vi "Send_Basic_Trajectory.vi"(8 "error in (no error)":errorcluster, 10 "TrajectoryPoint":T1) -> (0 "error out":errorcluster)   [LabVIEW 2019]
uses:
  <vilib>/Utility/error.llb/Error Cluster From Error Code.vi
  <vilib>/ErrorRing/Error Ring.xnode
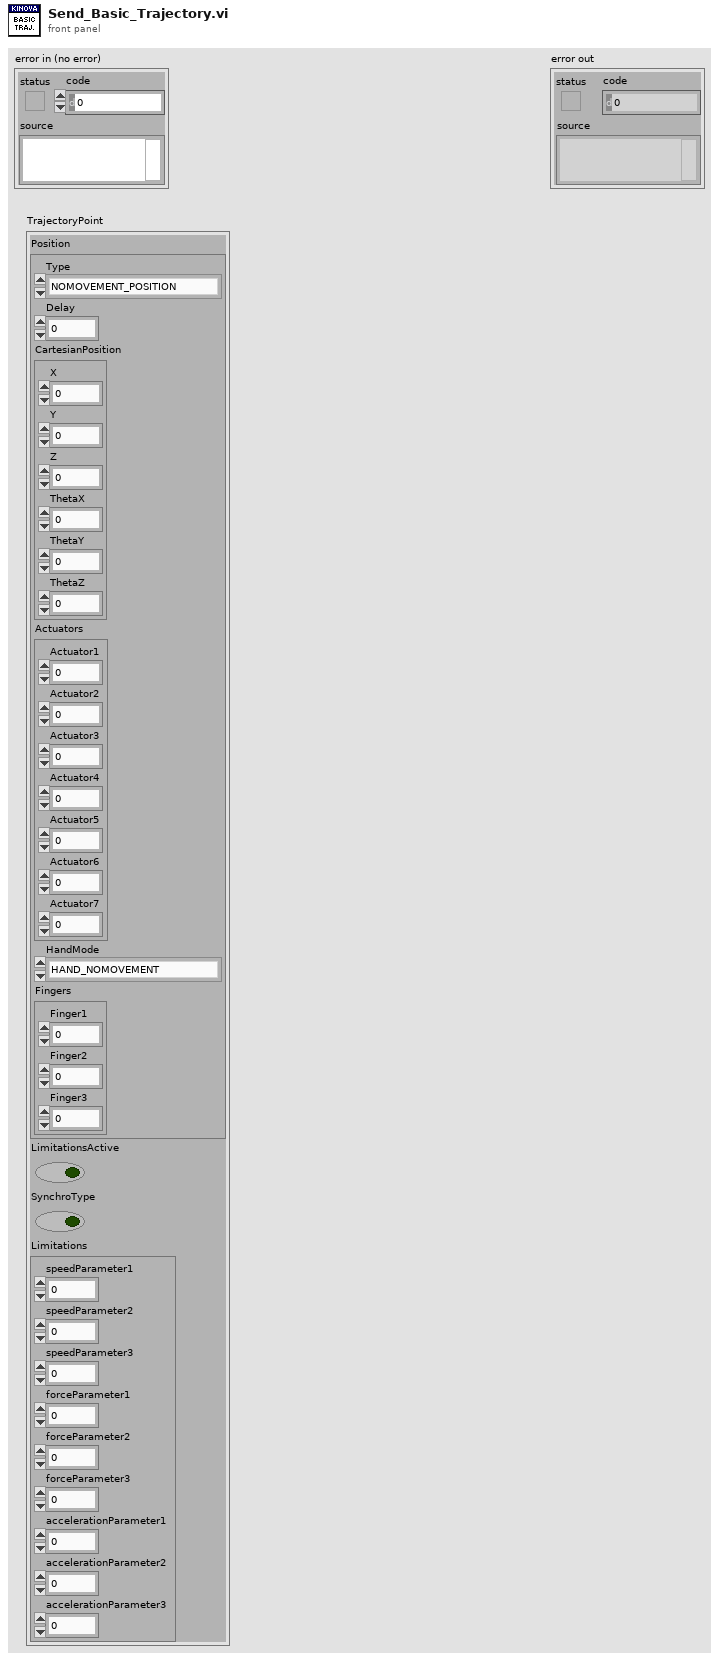
[diagram p1: front panel]
types:
  T1 = cluster{"Position":cluster{"Type":enum16{"NOMOVEMENT_POSITION", "CARTESIAN_POSITION", "ANGULAR_POSITION", "RETRACTED", "PREDEFINED1", "PREDEFINED2", "PREDEFINED3", "CARTESIAN_VELOCITY", "ANGULAR_VELOCITY", "PREDEFINED4", "PREDEFINED5", "ANY_TRAJECTORY", "TIME_DELAY"}, "Delay":sgl, "CartesianPosition":cluster{"X":sgl, "Y":sgl, "Z":sgl, "ThetaX":sgl, "ThetaY":sgl, "ThetaZ":sgl}, "Actuators":cluster{"Actuator1":sgl, "Actuator2":sgl, "Actuator3":sgl, "Actuator4":sgl, "Actuator5":sgl, "Actuator6":sgl, "Actuator7":sgl}, "HandMode":enum16{"HAND_NOMOVEMENT", "POSITION_MODE", "VELOCITY_MODE", "NO_FINGER", "ONE_FINGER", "TWO_FINGERS", "THREE_FINGERS"}, "Fingers":cluster{"Finger1":sgl, "Finger2":sgl, "Finger3":sgl}}, "LimitationsActive":bool, "SynchroType":bool, "Limitations":cluster{"speedParameter1":sgl, "speedParameter2":sgl, "speedParameter3":sgl, "forceParameter1":sgl, "forceParameter2":sgl, "forceParameter3":sgl, "accelerationParameter1":sgl, "accelerationParameter2":sgl, "accelerationParameter3":sgl}}
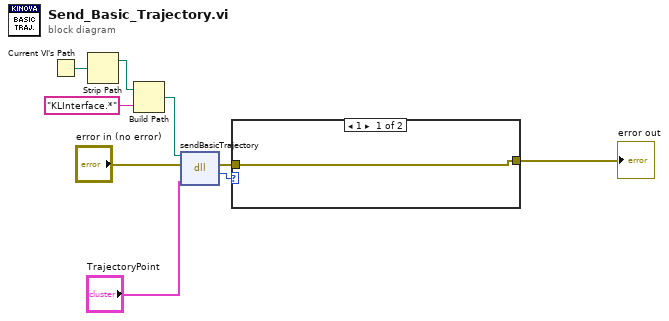
[diagram p0: block diagram]
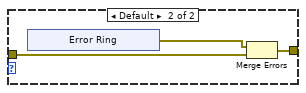
[diagram p2: hidden frame]
diagram:
  n1 = Current VI's Path() -> (path=w7:path)
  n2 = Strip Path(path=w7) -> (stripped path=w6:path)  [unwired: 1 out]
  n3 = Build Path(base path=w6, name or relative path="KLInterface.*") -> (appended path=w1:path)
  n4 = dll-call lib="C:/Users/mcjssdcc/source/repos/Kinova Labview Interface/Debug/KLInterface.dll" fn="sendBasicTrajectory"(path in=w1, error in="error in (no error)", "point"="TrajectoryPoint") -> (error out=w5:errorcluster, "return type"=w4:i32)  [unwired: 2 in, 1 out]
  n5 = case shown="1" w4 {
    tunnel: [w10 w12] -> w3
    tunnel: w5 -> [w10 w11]
    frame 1 {
    }
    frame Default {
      n6 = xnode "Error Ring"() -> ("error out"=w13:errorcluster)
      n7 = Merge Errors(w13, w11) -> (w12:errorcluster)
    }
  }
  "error out" <- w3
